vi "Pneumatic Control Loop.vi"(6 "reinit":bool, 10 "Process Variable":dbl, 11 "High Pressure":bool) -> (0 "Finished":bool, 2 "Release":bool, 3 "High Pressure":bool)   [LabVIEW 2013]
uses:
  Common Code/Change Detect Boolean.vi
  Robot Global Data.vi
  <vilib>/addons/control/pid/NI_PID_pid.lvlib
  <vilib>/addons/control/pid/pid.llb/PID (DBL).vi
panel:
  out "Force Blink":bool
  in  "Charts Enabled":bool
  out "PID Output":T1(graph)
  out "PID Inputs":T2(graph)
  in  "Setpoint":dbl
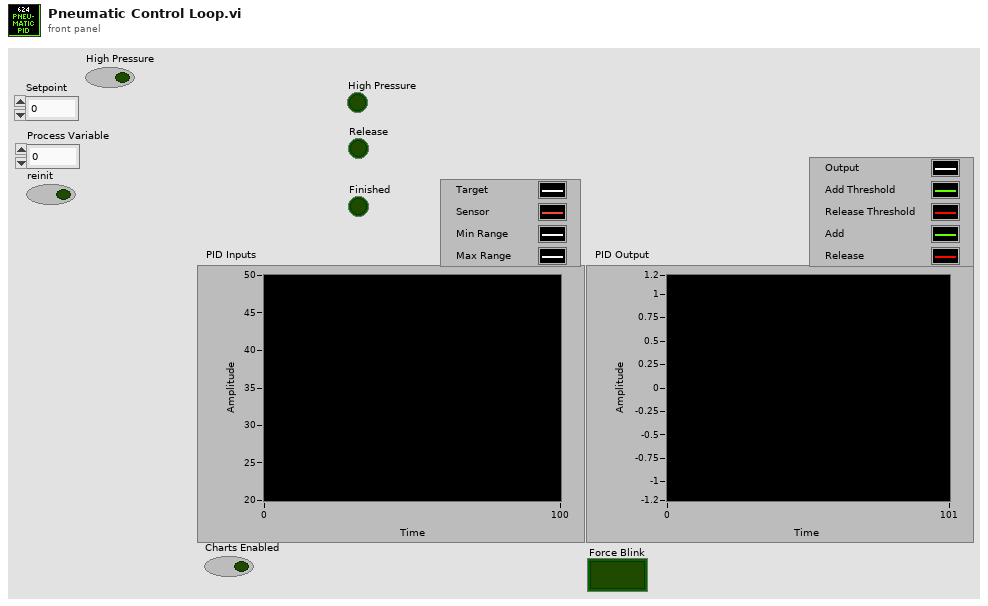
[diagram p1: front panel]
types:
  T1 = cluster{"output":dbl, "output high":dbl, "output low":dbl, "f":dbl, "f":dbl}
  T2 = cluster{"Setpoint":dbl, "Process Variable":dbl, "Numeric":dbl, dbl}
  T3 = cluster{"Setpoint":dbl, "Process Variable":dbl, dbl, dbl}
  T4 = cluster{"proportional gain (Kc)":dbl, "integral time (Ti, min)":dbl, "derivative time (Td, min)":dbl}
  T5 = typedef "Dashboard UDP Packet.ctl" = cluster{"Camera":T6, "Gyro":T7, "Encoder":T8, "Auto Shift":T9, "Auton":T10, "Drive/Ramp X":dbl, "Drive/Ramp Y":dbl, "Drive/Battery Cutoff":dbl, "Pressure/Compressor Min Voltage":dbl, "Pressure/Compressor Delay":dbl, "Controller/Strafe Correction":bool, "Shooter":T11, "Rollers":T12, "Abort":bool, "Finish":bool}
  T6 = typedef "Camera Controls.ctl" = cluster{"Camera/View Angle X":dbl, "Camera/Goal Track Timeout":dbl, "Camera/View Angle Y":dbl, "Camera/Goal Exposure":dbl, "Camera/Vision Receive Timeout":dbl, "Camera/Offset 1":dbl, "Camera/Offset 2":dbl}
  T7 = typedef "Gyro Controls.ctl" = cluster{"Gyro/Steer Close PID P":dbl, "Gyro/Steer Close PID I":dbl, "Gyro/Steer Close PID D":dbl, "Gyro/Steer Close PID min":dbl, "Gyro/Steer Close PID max":dbl, "Gyro/Steer PID P":dbl, "Gyro/Steer PID I":dbl, "Gyro/Steer PID D":dbl, "Gyro/Steer PID min":dbl, "Gyro/Angle Tolerance":dbl, "Gyro/Steer PID max":dbl, "Gyro/Steer Closeness Threshold":dbl}
  T8 = typedef "Encoder Controls.ctl" = cluster{"Encoders/Reset":bool, "Encoders/Omni Constant":dbl, "Encoders/Omni Tick Constant":dbl, "Encoders/Left Constant":dbl, "Encoders/Right Constant":dbl, "Encoders/Right Tick Constant":dbl}
  T9 = typedef "Auto Shift Controls.ctl" = cluster{"AutoShift/Upshift Throttle Accel":dbl, "AutoShift/Speed Threshold":dbl, "AutoShift/Upshift Throttle":dbl, "AutoShift/Upshift Accel":dbl, "AutoShift/Downshift Accel":dbl, "AutoShift/Downshift Throttle":dbl, "AutoShift/Delay":dbl, "AutoShift/Enabled":bool}
  T10 = typedef "Auton Controls.ctl" = cluster{"Auton/Left Shoot X-Coord":dbl, "Auton/Right Shoot X-Coord":dbl, "DistDrive/Distance Stop Threshold":dbl, "DistDrive/Max Stop Speed":dbl, "Auton/Back Piston Time":dbl, "Auton/Manual Hot":bool, "Auton/Manual Hot Right":bool, "Auton/X Distance PID max":dbl, "Auton/X Distance PID min":dbl, "Auton/X Distance PID P":dbl, "Auton/X Distance PID I":dbl, "Auton/X Distance PID D":dbl, "Auton/Y Distance PID max":dbl, "Auton/Y Distance PID min":dbl, "Auton/Y Distance PID P":dbl, "Auton/Y Distance PID I":dbl, "Auton/Y Distance PID D":dbl}
  T11 = typedef "Shooter Controls.ctl" = cluster{"Shooter/Reset Time":dbl, "Shooter/Release Delay":dbl, "Shooter/Pressure Steady Time":dbl, "Shooter/Misfire Delay":dbl, "Shooter/Ball Settle Time":dbl, "Shooter/Line IR Delay":dbl, "Pressure/Upper PSI Time":dbl, "Pressure/Lower PSI Time":dbl, "Shooter/Punch Delay":dbl, "Shooter/Target Pressure":dbl, "Pressure/Line B":dbl, "Pressure/Line M":dbl, "Pressure/Shooter M":dbl, "Pressure/Shooter B":dbl}
  T12 = typedef "Roller Controls.ctl" = cluster{"Roller/Load IRs Verify Time":dbl, "Roller/Center IR Latch Time":dbl, "Roller/Speed Front":dbl, "Roller/Speed Back":dbl, "Roller/Entry Timeout":dbl, "Roller/To Center Timeout":dbl, "Roller/Sustain Time":dbl, "Roller/Verify Center Time":dbl}
  T13 = cluster{"output":dbl, "output":dbl, "output":dbl, "f":dbl, "f":dbl}
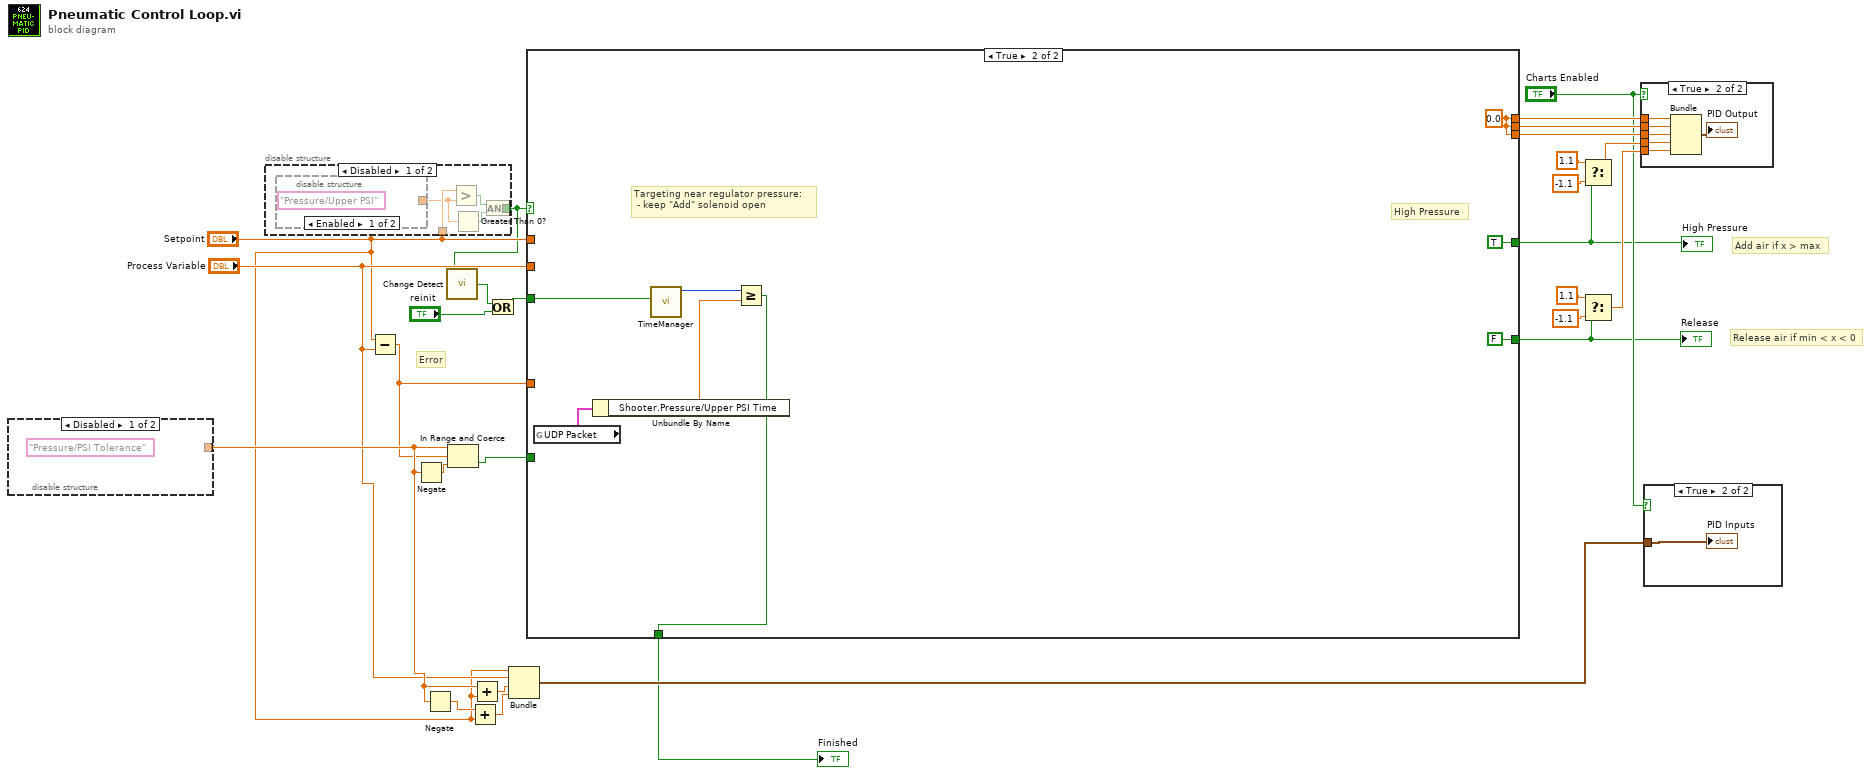
[diagram p0: block diagram]
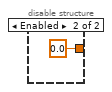
[diagram p2: hidden frame]
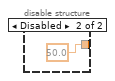
[diagram p3: hidden frame]
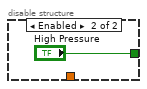
[diagram p4: hidden frame]
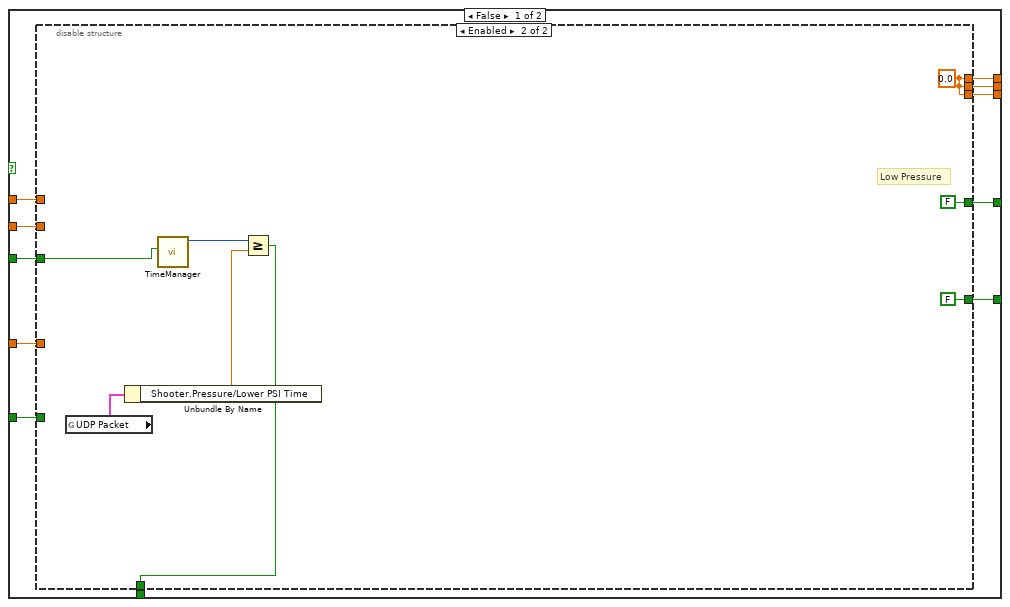
[diagram p5: hidden frame]
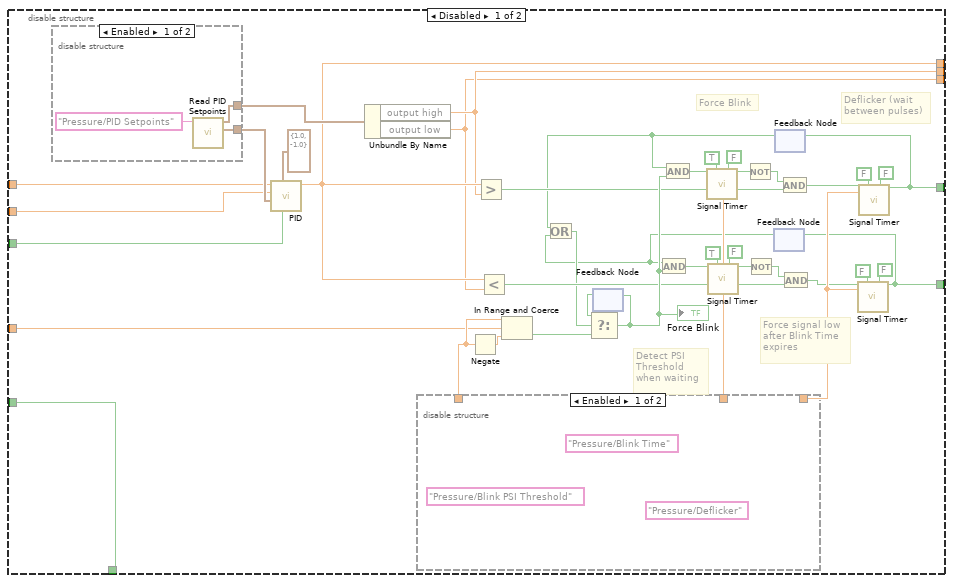
[diagram p6: hidden frame]
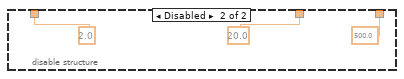
[diagram p7: hidden frame]
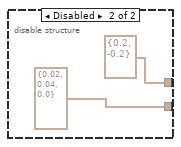
[diagram p8: hidden frame]
diagram:
  # "Error"
  # "Release air if min < x < 0"
  # "Add air if x > max"
  n1 = disable-structure shown="Disabled" {
    disable-tunnel: [_ 0.0 ("Numeric")] -> w13
    frame Disabled {
      w28 = "Pressure/PSI Tolerance" ("Name")
    }
    frame Enabled {
    }
  }
  n2 = disable-structure shown="Disabled" {
    disable-tunnel: "Setpoint" -> [w34 _]
    disable-tunnel: [w30 "High Pressure"] -> w1
    frame Disabled {
      n3 = disable-structure shown="Enabled" {
        disable-tunnel: [_ 50.0 ("Setpoint")] -> w31
        frame Enabled {
          w35 = "Pressure/Upper PSI" ("Name")
        }
        frame Disabled {
        }
      }
      n4 = Greater?(x=w34, y=w31) -> (0:w32:bool)
      n5 = Greater Than 0?(x=w31) -> (x > 0?=w33:bool)
      n6 = And(x=w32, y=w33) -> (x .and. y?=w30:bool)
    }
    frame Enabled {
    }
  }
  n7 = Subtract(x="Setpoint", y="Process Variable") -> (x-y=w9:dbl)
  n8 = Negate(x=w13) -> (-x=w27:dbl)
  n9 = Negate(x=w13) -> (-x=w14:dbl)
  n10 = call-poly "Change Detect.vi"("In"=w1) -> ("Changed?"=w2:bool)
  n11 = In Range and Coerce(upper limit=w13, x=w9, lower limit=w27) -> (In Range?=w5:bool)  [unwired: 1 out]
  n12 = Add(x=w14, y="Setpoint") -> (x+y=w15:dbl)
  n13 = Add(x=w13, y="Setpoint") -> (x+y=w12:dbl)
  n14 = Or(x=w2, y="reinit") -> (x .or. y?=w3:bool)
  n15 = Bundle("Setpoint"="Setpoint", "Process Variable"="Process Variable", w12, w15) -> (w16:T3)  [unwired: 1 in]
  n16 = case shown="True" w1 {
    tunnel: [w48 w117] -> w26
    tunnel: [w47 w117] -> w25
    tunnel: [w46 w117] -> w24
    tunnel: [w45 FALSE ("Filtered Output")] -> w11
    tunnel: [w44 TRUE ("Filtered Output")] -> w10
    tunnel: w9 -> [w43 _]
    tunnel: "Setpoint" -> [w42 _]
    tunnel: "Process Variable" -> [w41 _]
    tunnel: [w39 w114] -> w6
    tunnel: w5 -> [w38 _]
    tunnel: w3 -> [w40 w116]
    frame False {
      n17 = disable-structure shown="Enabled" {
        disable-tunnel: [w86 w111] -> w48
        disable-tunnel: [w85 w111] -> w47
        disable-tunnel: [w84 w111] -> w46
        disable-tunnel: [w70 FALSE ("Filtered Output")] -> w45
        disable-tunnel: [w68 FALSE ("Filtered Output")] -> w44
        disable-tunnel: w43 -> [w61 _]
        disable-tunnel: w42 -> [w60 _]
        disable-tunnel: w41 -> [w59 _]
        disable-tunnel: w40 -> [w50 w107]
        disable-tunnel: [w49 w106] -> w39
        disable-tunnel: w38 -> [w49 _]
        frame Disabled {
          # "Force signal low\nafter Blink Time \nexpires"
          # "Deflicker (wait\nbetween pulses)"
          # "Force Blink"
          # "Detect PSI\nThreshold\nwhen waiting"
          n18 = disable-structure shown="Enabled" {
            disable-tunnel: [w101 T4 {"proportional gain (Kc)"=0.02, "integral time (Ti, min)"=0.04, "derivative time (Td, min)"=0.0} ("PID gains")] -> w89
            disable-tunnel: [w99 cluster{"output high":dbl, "output low":dbl} {"output high"=0.2, "output low"=-0.2} ("output range")] -> w87
            frame Enabled {
              n19 = call "Read PID Setpoints.vi"("SD Name"="Pressure/PID Setpoints" ("string")) -> ("PID gains"=w101:T4, "output range"=w99:cluster{"output high":dbl, "output low":dbl})  [unwired: 9 in]
            }
            frame Disabled {
            }
          }
          n20 = call-poly <vilib>:"PID.vi"("reinitialize? (F)"=w50, "output range"=cluster{"output high":dbl, "output low":dbl} {"output high"=1.0, "output low"=-1.0}, "PID gains"=w89, "process variable"=w59, "setpoint"=w60) -> ("output"=w86:dbl)  [unwired: 5 in, 1 out]
          n21 = Unbundle By Name(w87) -> ("output high"=w85:dbl, "output low"=w84:dbl)
          n22 = disable-structure shown="Enabled" {
            disable-tunnel: [w94 500.0 ("Interval")] -> w79
            disable-tunnel: [w92 20.0 ("Interval")] -> w66
            disable-tunnel: [w90 2.0 ("Numeric")] -> w62
            frame Enabled {
              w91 = "Pressure/Blink PSI Threshold" ("Name")
              w93 = "Pressure/Blink Time" ("Name")
              w95 = "Pressure/Deflicker" ("Name")
            }
            frame Disabled {
            }
          }
          n23 = Negate(x=w62) -> (-x=w63:dbl)
          n24 = Greater?(x=w86, y=w85) -> (0:w55:bool)
          n25 = Less?(x=w86, y=w84) -> (x < y?=w54:bool)
          n26 = In Range and Coerce(upper limit=w62, x=w61, lower limit=w63) -> (In Range?=w58:bool)  [unwired: 1 out]
          n27 = feedback #1() -> (w56:bool)  [unwired: 1 in]
          n28 = feedback #2() -> (w51:bool)  [unwired: 1 in]
          n29 = feedback #3() -> (w52:bool)  [unwired: 1 in]
          n30 = Or(x=w52, y=w51) -> (x .or. y?=w53:bool)
          n31 = Select(t=w56, s=w53, f=w58) -> (s? t:f=w57:bool)
          "Force Blink" <- w57
          n32 = feedback-in #1(w57) -> ()
          n33 = And(x=w51, y=w57) -> (x .and. y?=w65:bool)
          n34 = And(x=w52, y=w57) -> (x .and. y?=w64:bool)
          n35 = call "Signal Timer.vi"("Input"=w64, "Edge"=TRUE, "Interval"=w66, "Pull"=FALSE ("Edge")) -> ("Filtered Output"=w76:bool)  [unwired: 11 in]
          n36 = call "Signal Timer.vi"("Input"=w65, "Edge"=TRUE, "Interval"=w66, "Pull"=FALSE ("Edge")) -> ("Filtered Output"=w73:bool)  [unwired: 11 in]
          n37 = Not(x=w76) -> (.not. x?=w75:bool)
          n38 = Not(x=w73) -> (.not. x?=w74:bool)
          n39 = And(x=w75, y=w55) -> (x .and. y?=w67:bool)
          n40 = And(x=w74, y=w54) -> (x .and. y?=w69:bool)
          n41 = call "Signal Timer.vi"("Input"=w69, "Edge"=FALSE, "Interval"=w79, "Pull"=FALSE ("Edge")) -> ("Filtered Output"=w70:bool)  [unwired: 11 in]
          n42 = feedback-in #2(w70) -> ()
          n43 = call "Signal Timer.vi"("Input"=w67, "Edge"=FALSE, "Interval"=w79, "Pull"=FALSE ("Edge")) -> ("Filtered Output"=w68:bool)  [unwired: 11 in]
          n44 = feedback-in #3(w68) -> ()
        }
        frame Enabled {
          w111 = 0.0 ("output")
          # "Low Pressure"
          n45 = global read "Robot Global Data.vi" "UDP Packet"() -> (w104:T5)
          n46 = Unbundle By Name(w104) -> ("Shooter.Pressure/Lower PSI Time"=w105:dbl)
          n47 = call "TimeManager.vi"("Reset?"=w107) -> ("Time Since Reset"=w108:u32)  [unwired: 9 in, 1 out]
          n48 = Greater Or Equal?(x=w108, y=w105) -> (x >= y?=w106:bool)
        }
      }
    }
    frame True {
      w117 = 0.0 ("output")
      # "High Pressure"
      # "Targeting near regulator pressure: \n - keep \"Add\" solenoid open"
      n49 = global read "Robot Global Data.vi" "UDP Packet"() -> (w112:T5)
      n50 = Unbundle By Name(w112) -> ("Shooter.Pressure/Upper PSI Time"=w113:dbl)
      n51 = call "TimeManager.vi"("Reset?"=w116) -> ("Time Since Reset"=w115:u32)  [unwired: 9 in, 1 out]
      n52 = Greater Or Equal?(x=w115, y=w113) -> (x >= y?=w114:bool)
    }
  }
  "Finished" <- w6
  "High Pressure" <- w10
  "Release" <- w11
  n53 = Select(t=1.1, s=w10, f=-1.1) -> (s? t:f=w21:dbl)
  n54 = Select(t=1.1, s=w11, f=-1.1) -> (s? t:f=w18:dbl)
  n55 = case shown="True" "Charts Enabled" {
    tunnel: w26 -> [_ w125]
    tunnel: w25 -> [_ w124]
    tunnel: w24 -> [_ w123]
    tunnel: w21 -> [_ w121]
    tunnel: w18 -> [_ w120]
    frame False {
    }
    frame True {
      n56 = Bundle("output"=w125, "output"=w124, "output"=w123, "f"=w121, "f"=w120) -> (→"PID Output":T13)  [unwired: 1 in]
    }
  }
  n57 = case shown="True" "Charts Enabled" {
    tunnel: w16 -> [_ w126]
    frame False {
    }
    frame True {
      "PID Inputs" <- w126
    }
  }
